vi "KeepStraight.vi"(6 "GyroData":T1, 8 "RightSpdIn":dbl, 9 "FirstTime?":bool, 10 "MtrDir":dbl, 11 "LeftSpdIn":dbl) -> (0 "RightSpdOut":dbl, 3 "LeftSpdOut":dbl)   [LabVIEW 2017]
uses:
  KeepStraightBoost.ctl
  2ea6bddf-f66a-4e8e-b269-0962688d1234.vi
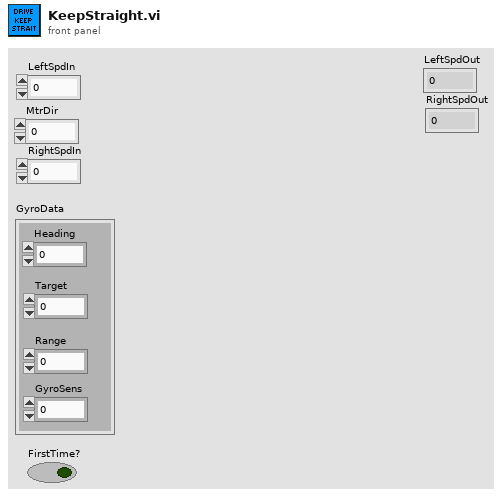
[diagram p1: front panel]
types:
  T1 = cluster{"Heading":dbl, "Target":dbl, "Range":dbl, "GyroSens":dbl}
  T2 = typedef "KeepStraightBoost.ctl" = string
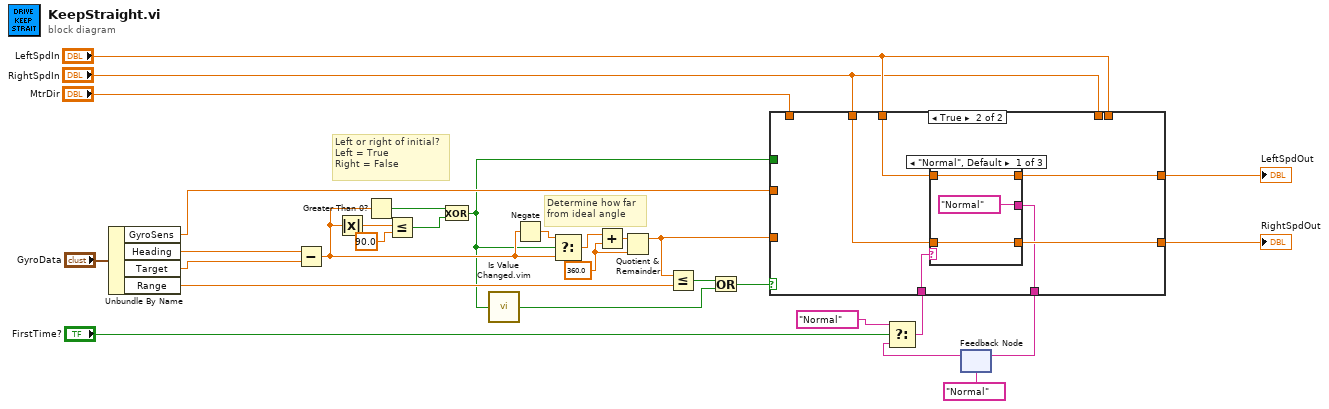
[diagram p0: block diagram]
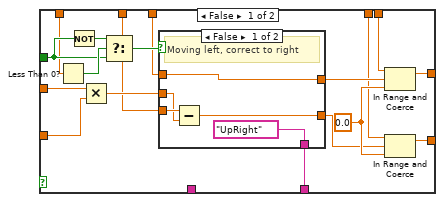
[diagram p2: hidden frame]
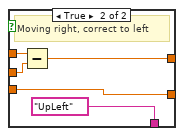
[diagram p3: hidden frame]
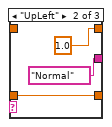
[diagram p4: hidden frame]
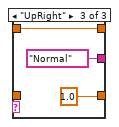
[diagram p5: hidden frame]
diagram:
  w24 = 360.0 ("value")
  # "Determine how far\nfrom ideal angle"
  # "Left or right of initial?\nLeft = True\nRight = False"
  n1 = Unbundle By Name("GyroData") -> ("GyroSens"=w16:dbl, "Heading"=w14:dbl, "Target"=w15:dbl, "Range"=w13:dbl)
  n2 = Subtract(x=w14, y=w15) -> (x-y=w22:dbl)
  n3 = Absolute Value(x=w22) -> (abs(x)=w28:dbl)
  n4 = Greater Than 0?(x=w22) -> (x > 0?=w30:bool)
  n5 = Less Or Equal?(x=w28, y=90.0) -> (x <= y?=w29:bool)
  n6 = Exclusive Or(1:w29, 2:w30) -> (0:w4:bool)
  n7 = call "Is Value Changed.vim"("value"=w4) -> ("changed or first call?"=w2:bool)
  n8 = Negate(x=w22) -> (-x=w23:dbl)
  n9 = Select(t=w23, s=w4, f=w22) -> (s? t:f=w25:dbl)
  n10 = Add(x=w25, y=w24) -> (x+y=w26:dbl)
  n11 = Quotient & Remainder(x=w26, y=w24) -> (x-y*floor(x/y)=w21:dbl)  [unwired: 1 out]
  n12 = Less Or Equal?(x=w21, y=w13) -> (x <= y?=w3:bool)
  n13 = Or(x=w3, y=w2) -> (x .or. y?=w1:bool)
  n14 = feedback #1(T2 "Normal" ("Combo Box")) -> (w8:T2)
  n15 = Select(t=T2 "Normal" ("Combo Box"), s="FirstTime?", f=w8) -> (s? t:f=w5:T2)
  n16 = case shown="True" w1 {
    tunnel: w4 -> [w43 _]
    tunnel: w16 -> [w39 _]
    tunnel: w21 -> [w38 _]
    tunnel: [w46 w64] -> w19
    tunnel: [w45 w63] -> w18
    tunnel: "MtrDir" -> [w40 _]
    tunnel: "LeftSpdIn" -> [w35 w62]
    tunnel: "RightSpdIn" -> [w34 w61]
    tunnel: "RightSpdIn" -> [w33 _]
    tunnel: "LeftSpdIn" -> [w32 _]
    tunnel: [w31 w59] -> w10
    tunnel: w5 -> [_ w60]
    frame False {
      w47 = 0.0 ("lower limit")
      n17 = Less Than 0?(x=w40) -> (x < 0?=w44:bool)
      n18 = Not(x=w43) -> (.not. x?=w42:bool)
      n19 = Multiply(x=w39, y=w38) -> (x*y=w48:dbl)
      n20 = Select(t=w42, s=w44, f=w43) -> (s? t:f=w41:bool)
      n21 = case shown="False" w41 {
        tunnel: w35 -> [w53 w57]
        tunnel: w48 -> [w51 w58]
        tunnel: [w50 w55] -> w37
        tunnel: [w53 w56] -> w36
        tunnel: w34 -> [w52 w55]
        tunnel: [T2 "UpRight" ("Combo Box") T2 "UpLeft" ("Combo Box")] -> w31
        frame False {
          # "Moving left, correct to right"
          n22 = Subtract(x=w52, y=w51) -> (x-y=w50:dbl)
        }
        frame True {
          # "Moving right, correct to left"
          n23 = Subtract(x=w57, y=w58) -> (x-y=w56:dbl)
        }
      }
      n24 = In Range and Coerce(upper limit=w32, x=w36, lower limit=w47) -> (coerced(x)=w46:dbl)  [unwired: 1 out]
      n25 = In Range and Coerce(upper limit=w33, x=w37, lower limit=w47) -> (coerced(x)=w45:dbl)  [unwired: 1 out]
    }
    frame True {
      n26 = case shown="\"Normal\", Default" w60 {
        tunnel: w62 -> [w66 _ w73]
        tunnel: [w67 w70 1.0 ("x")] -> w63
        tunnel: w61 -> [w67 w70 _]
        tunnel: [w66 1.0 ("x") w73] -> w64
        tunnel: [T2 "Normal" ("Combo Box") T2 "Normal" ("Combo Box") T2 "Normal" ("Combo Box")] -> w59
        frame "Normal", Default {
        }
        frame "UpLeft" {
        }
        frame "UpRight" {
        }
      }
    }
  }
  "LeftSpdOut" <- w19
  "RightSpdOut" <- w18
  n27 = feedback-in #1(w10) -> ()
